vi "Launch-deposition.vi"(8 "error in (no error)":errorcluster, 11 "Object ref in":T1) -> (0 "error out":errorcluster, 3 "Object ref out":T1)   [LabVIEW 2013, in "SLMControl.lvlib" / "SC-Main.lvclass"]
uses:
  SC-Main.lvclass
  Object-reference.ctl
  Client/Sources/Supported-modules.ctl
  Client/Sources/Supported-actions.ctl
  SC-Main.lvclass/SC-Main.ctl
  Read Client.vi
  Client/Sources/SC-Client.lvclass
  SA-SLMAPI/Sources/Action/Action.lvclass
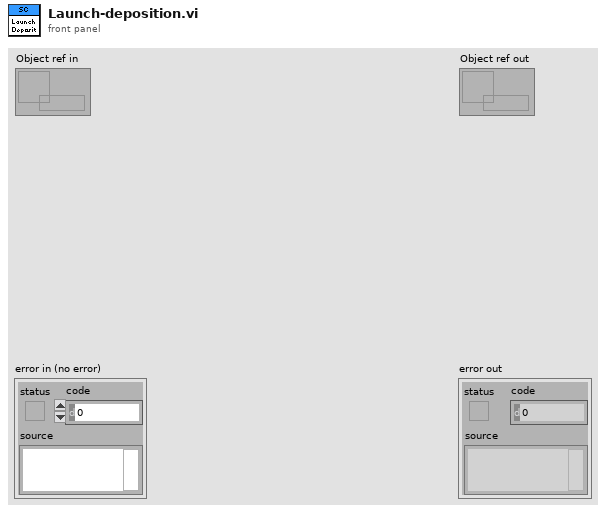
[diagram p1: front panel]
types:
  T1 = typedef "SLMControl.lvlib/SC-Main.lvclass/Object-reference.ctl" = refnum<data-value>
  T2 = typedef "SLMControl.lvlib/SC-Client.lvclass/Supported-actions.ctl" = enum16{"Idle", "Initialize", "Load settings", "Load file", "Activate", "Start", "Pause", "Stop", "Repeat", "Reset", "Exit"}
  T3 = typedef "SLMControl.lvlib/SC-Client.lvclass/Supported-modules.ctl" = enum16{"Server", "All", "SLMControl", "PowderDeposition", "StrategyParser", "CameraVision", "MaterialCharacterization", "StatusMonitor", "SLMSimulation", "LaserCharacterization"}
  T4 = typedef "SLMControl.lvlib/SC-Client.lvclass/Object-reference.ctl" = refnum<data-value>
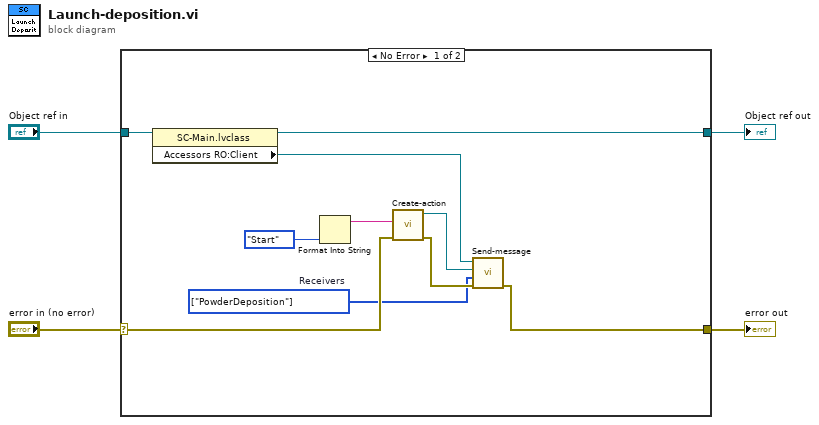
[diagram p0: block diagram]
diagram:
  n1 = case shown="No Error" "error in (no error)" {
    selector: "error in (no error)" -> [w8 w16]
    tunnel: [w10 w16] -> w3
    tunnel: [w13 w15] -> w1
    tunnel: "Object ref in" -> [w14 w15]
    frame No Error {
      w5 = T3[] [enum."PowderDeposition"] items=["Server", "All", "SLMControl", "PowderDeposition", "StrategyParser", "CameraVision", "MaterialCharacterization", "StatusMonitor", "SLMSimulation", "LaserCharacterization"]  # Receivers
      n2 = property class="SC-Main.lvclass"(reference=w14) -> (reference out=w13:T1, "Accessors RO:Client"=w11:T4)  [unwired: 1 in, 1 out]
      n3 = Format Into String(Supported-actions."Start" ("Action")) -> (resulting string=w6:string)  [unwired: 3 in, 1 out]
      n4 = call "Create-action.vi"("error in (no error)"=w8, "Action"=w6) -> ("error out"=w9:errorcluster, "Action out"=w12:refnum<class "Action.lvclass">)  [unwired: 8 in]
      n5 = call "Send-message.vi"("error in (no error)"=w9, "Receivers"=w5, "Message"=w12, "Client in"=w11) -> ("error out"=w10:errorcluster)  [unwired: 6 in, 1 out]
    }
    frame Error {
    }
  }
  "error out" <- w3
  "Object ref out" <- w1
